vi "error generator.vi"(5 "error (T)":bool=TRUE, 6 "error in":errorcluster, 7 "source":string="error generator.vi", 8 "append error message":string, 9 "error code (0)":i32) -> (0 "error out":errorcluster)   [LabVIEW 2013, in "NISE_CEF_TreeControl.lvlib"]
doc: "Converts an error or warning code to an error cluster. This VI is useful when you receive a return value from a shared library call or when you return user-defined error codes."
uses:
  NISE_CEF_TreeControl.lvlib
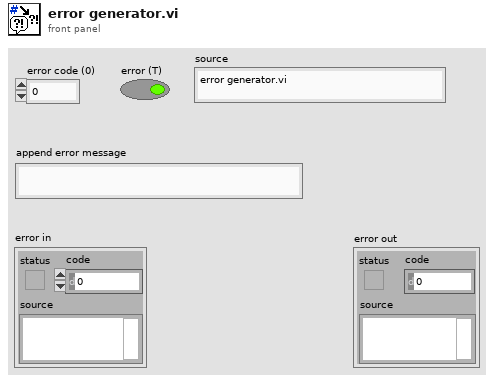
[diagram p1: front panel]
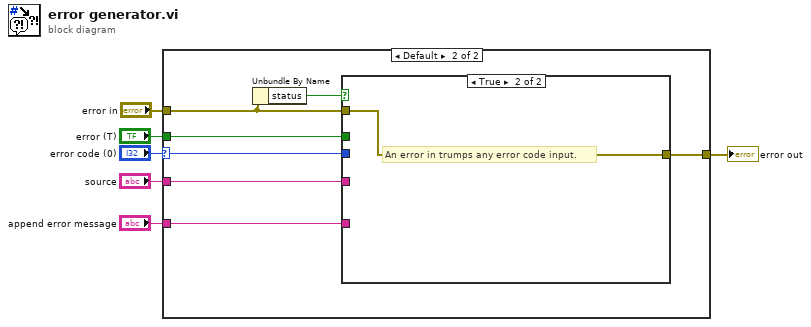
[diagram p0: block diagram]
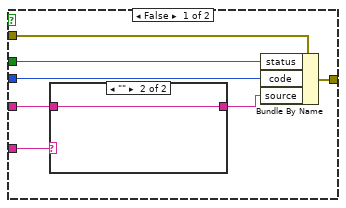
[diagram p3: hidden frame]
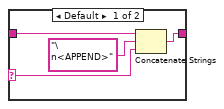
[diagram p4: hidden frame]
diagram:
  n1 = case shown="Default" "error code (0)" {
    selector: "error code (0)" -> [_ w13]
    tunnel: "error in" -> [w7 w9]
    tunnel: [w7 w14] -> w4
    tunnel: "source" -> [_ w12]
    tunnel: "append error message" -> [_ w11]
    tunnel: "error (T)" -> [_ w10]
    frame 0 {
      # "If the error code in equals zero, then propagate the error in cluster regardless of its value."
    }
    frame Default {
      n2 = Unbundle By Name(w9) -> ("status"=w8:bool)
      n3 = case shown="True" w8 {
        tunnel: [w20 w27] -> w14
        tunnel: w13 -> [w21 _]
        tunnel: w12 -> [w17 _]
        tunnel: w11 -> [w19 _]
        tunnel: w10 -> [w16 _]
        tunnel: w9 -> [w15 w27]
        frame False {
          n4 = case shown="\"\"" w19 {
            selector: w19 -> [w23 _]
            tunnel: [w22 w26] -> w18
            tunnel: w17 -> [w25 w26]
            frame Default {
              n5 = Concatenate Strings(w25, "\n<APPEND>" ("string"), w23) -> (w22:string)
            }
            frame "" {
            }
          }
          n6 = Bundle By Name(cluster=w15, "status"=w16, "code"=w21, "source"=w18) -> (w20:errorcluster)
        }
        frame True {
          # "An error in trumps any error code input."
        }
      }
    }
  }
  "error out" <- w4
